vi "Auto Nbr. STEP.vi"(8 "error in (no error)":errorcluster, 9 "index (col)":i32, 10 "STEP in":T1, 11 "STEPs In":T1[](array[typedef])) -> (0 "error out":errorcluster, 1 "Discarded?":bool, 3 "STEPs Out":T1[](array[typedef]))   [LabVIEW 2014, in "SeqLoop.lvlib"]
uses:
  SeqLoop.lvlib
  TypeDefs/STEP.ctl
  TypeDefs/LogicParsedExpression.ctl
  Mimico Display/TypeDefs/Mimic Data.ctl
  Mimico Display/TypeDefs/BG Image.ctl
  Mimico Display/TypeDefs/mObject.ctl
  Mimico Display/Mimico Display.lvlib
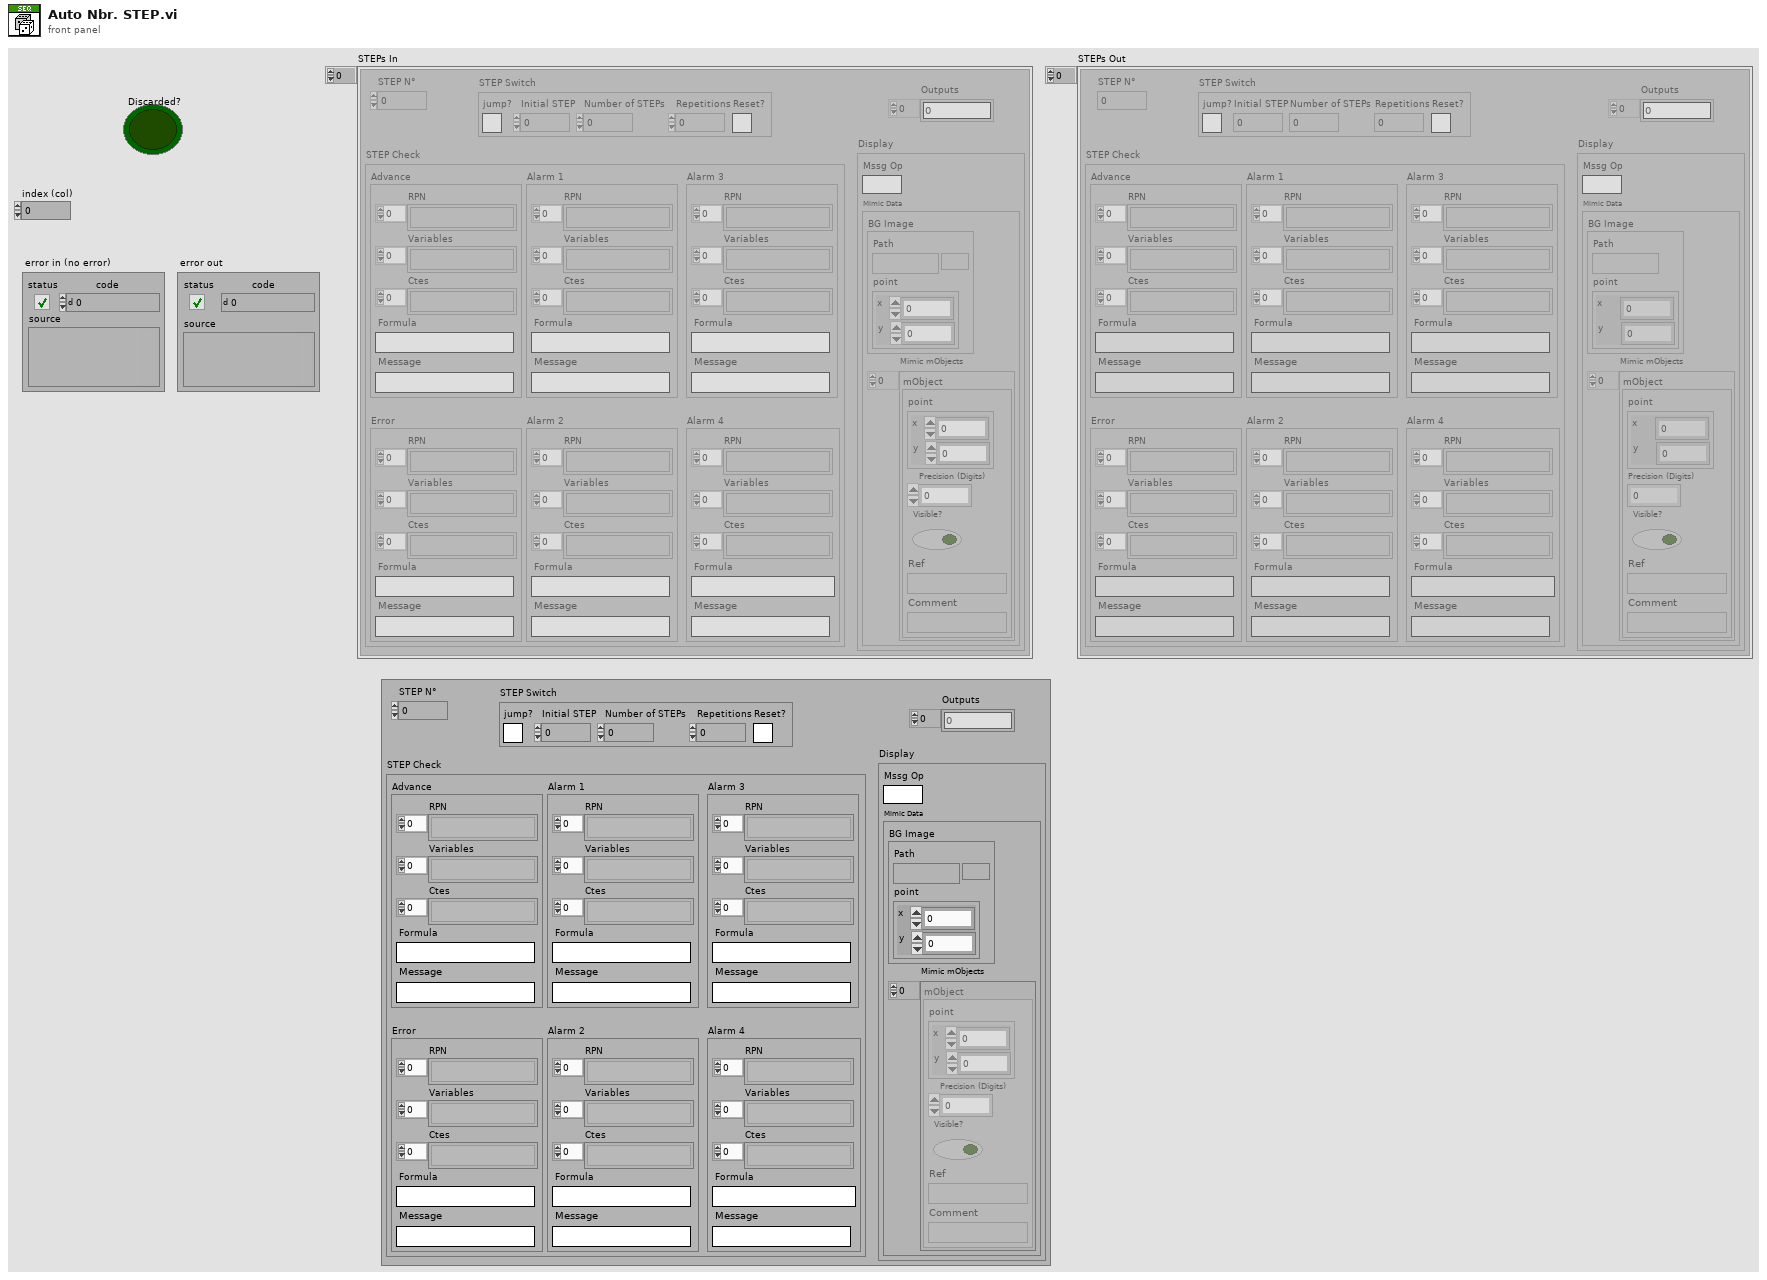
[diagram p1: front panel]
types:
  T1 = typedef "SeqLoop.lvlib/STEP.ctl" = cluster{"STEP N°":u32, "STEP Switch":cluster{"jump?":bool, "Initial STEP":u32, "Number of STEPs":u32, "Repetitions":u32, "Reset?":bool}, "Outputs":i32[], "STEP Check":cluster{"Advance":T2, "Error ":T2, "Alarm 1":T2, "Alarm 2":T2, "Alarm 3":T2, "Alarm 4":T2}, "Display":cluster{"Mssg Op":string, "Mimic Data":T3}}
  T2 = typedef "SeqLoop.lvlib/LogicParsedExpression.ctl" = cluster{"RPN ":string[], "Variables":string[], "Ctes":string[], "Formula":string, "Message":string}
  T3 = typedef "SeqLoop.lvlib/Mimico Display.lvlib/Mimic Data.ctl" = cluster{"BG Image":T4, "Mimic mObjects":T5[]}
  T4 = typedef "SeqLoop.lvlib/Mimico Display.lvlib/BG Image.ctl" = cluster{"Path":path, "point":cluster{"x":i16, "y":i16}}
  T5 = typedef "SeqLoop.lvlib/Mimico Display.lvlib/mObject.ctl" = cluster{"point":cluster{"x":i16, "y":i16}, "Precision (Digits)":i32, "Visible?":bool, "Ref":string, "Comment":string}
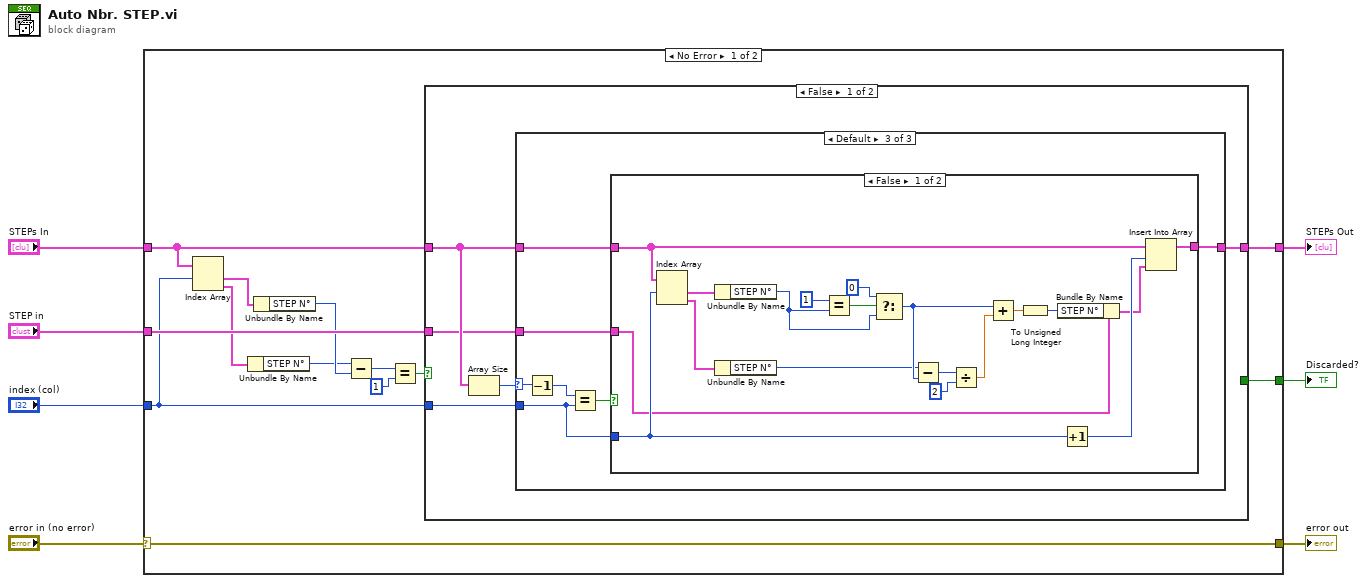
[diagram p0: block diagram]
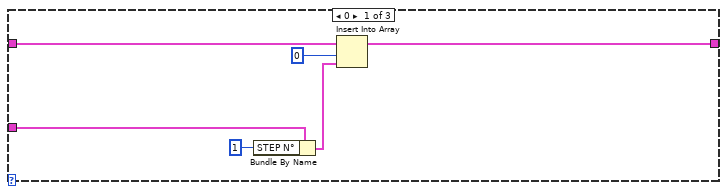
[diagram p2: hidden frame]
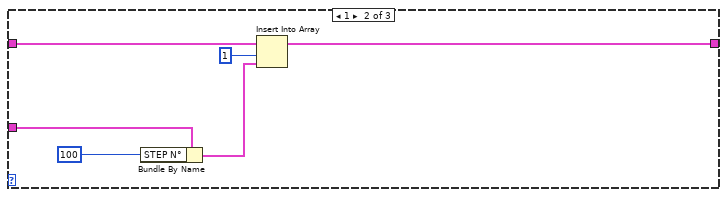
[diagram p3: hidden frame]
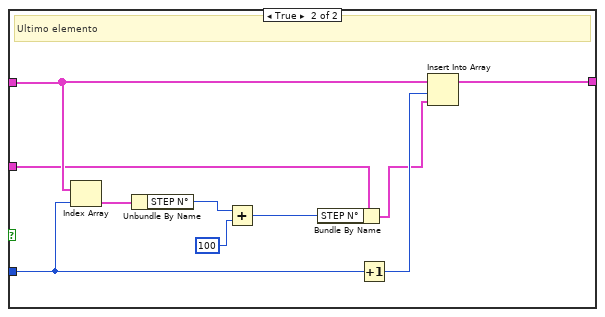
[diagram p4: hidden frame]
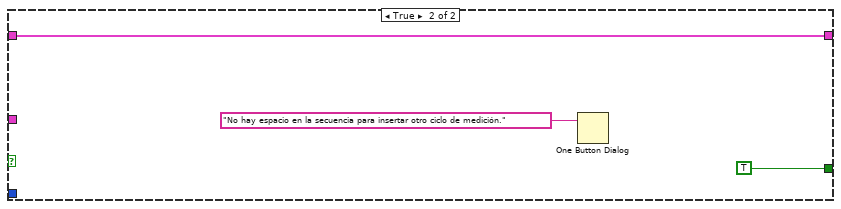
[diagram p5: hidden frame]
diagram:
  n1 = case shown="No Error" "error in (no error)" {
    selector: "error in (no error)" -> [w20 w78]
    tunnel: "STEPs In" -> [w18 w77]
    tunnel: "index (col)" -> [w12 _]
    tunnel: [w20 w78] -> w5
    tunnel: "STEP in" -> [w14 _]
    tunnel: [w19 w77] -> w2
    tunnel: [w13 _] -> w4
    frame No Error {
      n2 = Index Array(array=w18, index #1=w12) -> (element #1=w10:T1, element #2=w11:T1)  [unwired: 1 in]
      n3 = Unbundle By Name(w11) -> ("STEP N°"=w8:u32)
      n4 = Unbundle By Name(w10) -> ("STEP N°"=w9:u32)
      n5 = Subtract(x=w8, y=w9) -> (x-y=w16:u32)
      n6 = Equal?(x=w16, y=u32 1) -> (x = y?=w17:bool)
      n7 = case shown="False" w17 {
        tunnel: [w24 w76] -> w19
        tunnel: w18 -> [w23 w76]
        tunnel: w12 -> [w22 _]
        tunnel: w14 -> [w21 _]
        tunnel: [_ TRUE] -> w13
        frame False {
          n8 = Array Size(array=w23) -> (size(s)=w25:i32)
          n9 = case shown="Default" w25 {
            selector: w25 -> [_ _ w44]
            tunnel: w23 -> [w31 w37 w40]
            tunnel: w22 -> [_ _ w39]
            tunnel: w21 -> [w27 w34 w41]
            tunnel: [w30 w35 w38] -> w24
            frame 0 {
              n10 = Bundle By Name(cluster=w27, "STEP N°"=u32 1) -> (w26:T1)
              n11 = Insert Into Array(array=w31, index=0, new element=w26) -> (w30:T1[])
            }
            frame 1 {
              n12 = Bundle By Name(cluster=w34, "STEP N°"=u32 100) -> (w32:T1)
              n13 = Insert Into Array(array=w37, index=1, new element=w32) -> (w35:T1[])
            }
            frame Default {
              n14 = Decrement(x=w44) -> (x-1=w43:i32)
              n15 = Equal?(x=w43, y=w39) -> (x = y?=w42:bool)
              n16 = case shown="False" w42 {
                tunnel: w41 -> [w50 w68]
                tunnel: w40 -> [w54 w72]
                tunnel: w39 -> [w52 w70]
                tunnel: [w55 w71] -> w38
                frame False {
                  n17 = Index Array(array=w54, index #1=w52) -> (element #1=w48:T1, element #2=w46:T1)  [unwired: 1 in]
                  n18 = Unbundle By Name(w48) -> ("STEP N°"=w47:u32)
                  n19 = Unbundle By Name(w46) -> ("STEP N°"=w45:u32)
                  n20 = Equal?(x=u32 1 ("y"), y=w47) -> (x = y?=w62:bool)
                  n21 = Select(t=u32 0 ("y"), s=w62, f=w47) -> (s? t:f=w58:u32)
                  n22 = Subtract(x=w45, y=w58) -> (x-y=w60:u32)
                  n23 = Divide(x=w60, y=u32 2) -> (x/y=w57:dbl)
                  n24 = Add(x=w58, y=w57) -> (x+y=w56:dbl)
                  n25 = To Unsigned Long Integer(number=w56) -> (unsigned 32bit integer=w51:u32)
                  n26 = Bundle By Name(cluster=w50, "STEP N°"=w51) -> (w49:T1)
                  n27 = Increment(x=w52) -> (x+1=w53:i32)
                  n28 = Insert Into Array(array=w54, index=w53, new element=w49) -> (w55:T1[])
                }
                frame True {
                  # "Ultimo elemento"
                  n29 = Index Array(array=w72, index=w70) -> (element=w65:T1)
                  n30 = Unbundle By Name(w65) -> ("STEP N°"=w64:u32)
                  n31 = Add(x=w64, y=u32 100) -> (x+y=w66:u32)
                  n32 = Bundle By Name(cluster=w68, "STEP N°"=w66) -> (w67:T1)
                  n33 = Increment(x=w70) -> (x+1=w69:i32)
                  n34 = Insert Into Array(array=w72, index=w69, new element=w67) -> (w71:T1[])
                }
              }
            }
          }
        }
        frame True {
          n35 = One Button Dialog(message="No hay espacio en la secuencia para insertar otro ciclo de medición.") -> ()  [unwired: 1 in, 1 out]
        }
      }
    }
    frame Error {
    }
  }
  "error out" <- w5
  "Discarded?" <- w4
  "STEPs Out" <- w2
